vi "VImode.vi"() -> ()   [LabVIEW 2015]
panel:
  in  "Output Mode (Arbitrary Waveform)":i32(ring)=1 items=["Arbitrary Waveform"=1, "Arbitrary Sequence"=2]
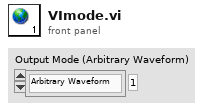
[diagram p1: front panel]
diagram:
